vi "TSNE.vi"(8 "error in":errorcluster) -> (0 "error out":errorcluster, 3 "out":refnum<class "TSNE.lvclass">)   [LabVIEW 2020]
doc: "t-distributed Stochastic Neighbor Embedding.\n\n t-SNE [1] is a tool to visualize high-dimensional data. It converts\n similarities between data points to joint probabilities and tries\n to minimize the Kullback-Leibler divergence between the joint\n probabilities of the low-dimensional embedding and the\n high-dimensional data. t-SNE has a cost function that is not convex,\n i.e. with different initializations we can get different results.\n\n It is highly recommended to use another dimensionality reduction\n method (e.g. PCA for dense data or TruncatedSVD for sparse data)\n to reduce the number of dimensions to a reasonable amount (e.g. 50)\n if the number of features is very high. This will suppress some\n noise and speed up the computation of pairwise distances between\n samples. For more tips see Laurens van der Maaten's FAQ [2].\n\n Read more in the :ref:`User Guide <t_sne>`.\n\n Parameters\n ----------\n n_components : int, default=2\n Dimension of the embedded space.\n\n perplexity : float, default=30.0\n The perplexity is related to the number of nearest neighbors that\n is used in other manifold learning algorithms. Larger datasets\n usually require a larger perplexity. Consider selecting a value\n between 5 and 50. Different values can result in significantly\n different results.\n\n early_exaggeration : float, default=12.0\n Controls how tight natural clusters in the original space are in\n the embedded space and how much space will be between them. For\n larger values, the space between natural clusters will be larger\n in the embedded space. Again, the choice of this parameter is not\n very critical. If the cost function increases during initial\n optimization, the early exaggeration factor or the learning rate\n might be too high.\n\n learning_rate : float, default=200.0\n The learning rate for t-SNE is usually in the range [10.0, 1000.0]. If\n the learning rate is too high, the data may look like a 'ball' with any\n point approximately equidistant from its nearest neighbours. If the\n learning rate is too low, most points may look compressed in a dense\n cloud with few outliers. If the cost function gets stuck in a bad local\n minimum increasing the learning rate may help.\n\n n_iter : int, default=1000\n Maximum number of iterations for the optimization. Should be at\n least 250.\n\n n_iter_without_progress : int, default=300\n Maximum number of iterations without progress before we abort the\n optimization, used after 250 initial iterations with early\n exaggeration. Note that progress is only checked every 50 iterations so\n this value is rounded to the next multiple of 50.\n\n .. versionadded:: 0.17\n parameter *n_iter_without_progress* to control stopping criteria.\n\n min_grad_norm : float, default=1e-7\n If the gradient norm is below this threshold, the optimization will\n be stopped.\n\n metric : str or callable, default='euclidean'\n The metric to use when calculating distance between instances in a\n feature array. If metric is a string, it must be one of the options\n allowed by scipy.spatial.distance.pdist for its metric parameter, or\n a metric listed in pairwise.PAIRWISE_DISTANCE_FUNCTIONS.\n If metric is \"precomputed\", X is assumed to be a distance matrix.\n Alternatively, if metric is a callable function, it is called on each\n pair of instances (rows) and the resulting value recorded. The callable\n should take two arrays from X as input and return a value indicating\n the distance between them. The default is \"euclidean\" which is\n interpreted as squared euclidean distance.\n\n init : {'random', 'pca'} or ndarray of shape (n_samples, n_components), default='random'\n Initialization of embedding. Possible options are 'random', 'pca',\n and a numpy array of shape (n_samples, n_components).\n PCA initialization cannot be used with precomputed distances and is\n usually more globally stable than random initialization.\n\n verbose : int, default=0\n Verbosity level.\n\n random_state : int, RandomState instance or None, default=None\n Determines the random number generator. Pass an int for reproducible\n results across multiple function calls. Note that different\n initializations might result in different local minima of the cost\n function. See :term: `Glossary <random_state>`.\n\n method : str, default='barnes_hut'\n By default the gradient calculation algorithm uses Barnes-Hut\n approximation running in O(NlogN) time. method='exact'\n will run on the slower, but exact, algorithm in O(N^2) time. The\n exact algorithm should be used when nearest-neighbor errors need\n to be better than 3%. However, the exact method cannot scale to\n millions of examples.\n\n .. versionadded:: 0.17\n Approximate optimization *method* via the Barnes-Hut.\n\n angle : float, default=0.5\n Only used if method='barnes_hut'\n This is the trade-off between speed and accuracy for Barnes-Hut T-SNE.\n 'angle' is the angular size (referred to as theta in [3]) of a distant\n node as measured from a point. If this size is below 'angle' then it is\n used as a summary node of all points contained within it.\n This method is not very sensitive to changes in this parameter\n in the range of 0.2 - 0.8. Angle less than 0.2 has quickly increasing\n computation time and angle greater 0.8 has quickly increasing error.\n\n n_jobs : int, default=None\n The number of parallel jobs to run for neighbors search. This parameter\n has no impact when ``metric=\"precomputed\"`` or\n (``metric=\"euclidean\"`` and ``method=\"exact\"``).\n ``None`` means 1 unless in a :obj:`joblib.parallel_backend` context.\n ``-1`` means using all processors. See :term:`Glossary <n_jobs>`\n for more details.\n\n .. versionadded:: 0.22\n\n square_distances : True or 'legacy', default='legacy'\n Whether TSNE should square the distance values. ``'legacy'`` means\n that distance values are squared only when ``metric=\"euclidean\"``.\n ``True`` means that distance values are squared for all metrics.\n\n .. versionadded:: 0.24\n Added to provide backward compatibility during deprecation of\n legacy squaring behavior.\n .. deprecated:: 0.24\n Legacy squaring behavior was deprecated in 0.24. The ``'legacy'``\n value will be removed in 1.1 (renaming of 0.26), at which point the\n default value will change to ``True``.\n\n Attributes\n ----------\n embedding_ : array-like of shape (n_samples, n_components)\n Stores the embedding vectors.\n\n kl_divergence_ : float\n Kullback-Leibler divergence after optimization.\n\n n_iter_ : int\n Number of iterations run.\n\n \nAvailable methods:\nFit\nFit Transform\nGet Attributes\nGet Params\nSet Params"
uses:
  TSNE.lvclass
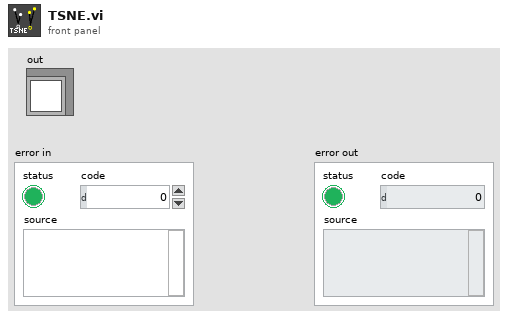
[diagram p1: front panel]
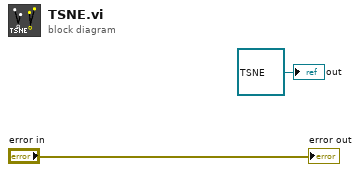
[diagram p0: block diagram]
diagram:
  "out" <- refnum<class "TSNE.lvclass"> refnum ("model")
  "error out" <- "error in"
